vi "Rollback Transaction.vi"(8 "error in":errorcluster, 11 "DB-SQLite in":refnum<class "DB-SQLite.lvclass">) -> (0 "error out":errorcluster, 3 "DB-SQLite out":refnum<class "DB-SQLite.lvclass">)   [LabVIEW 2022 SP3, in "hse-db-sqlite.lvlib" / "DB-SQLite.lvclass"]
doc: "Rollback the active transaction.\n\n____\nHAMPEL SOFTWARE ENGINEERING v1.4.0 (2023-12-19 09:52)"
uses:
  DB-SQLite.lvclass
  DB-SQLite.lvclass/DB-SQLite.ctl
  <vilib>/drjdpowell/SQLite Library/Transaction Helpers/Transaction.lvlib
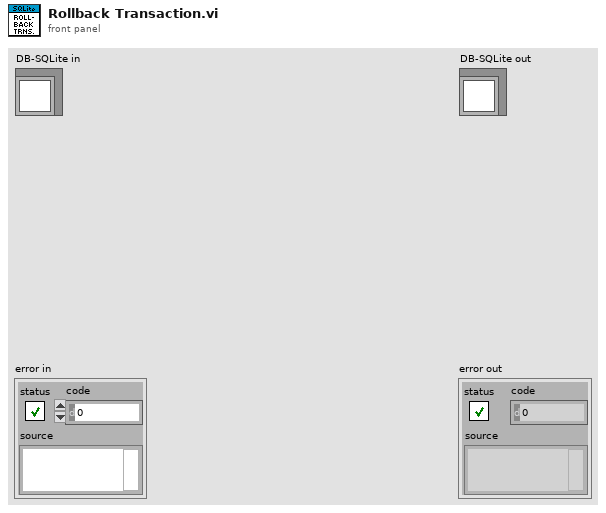
[diagram p1: front panel]
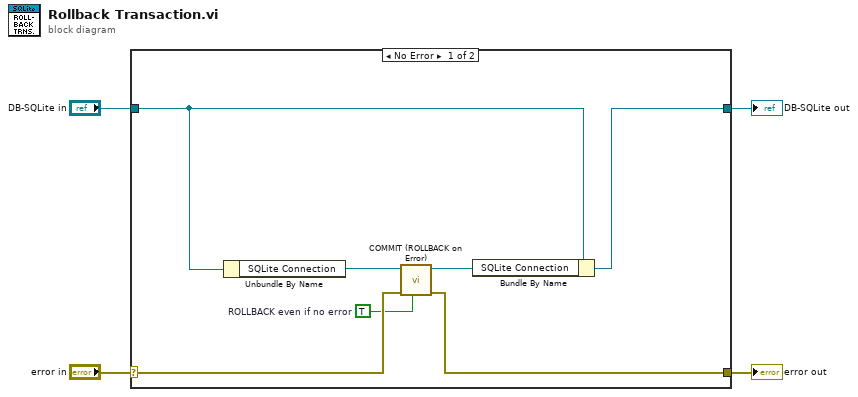
[diagram p0: block diagram]
diagram:
  n1 = case shown="No Error" "error in" {
    selector: "error in" -> [w9 w13]
    tunnel: [w6 w13] -> w3
    tunnel: [w10 w12] -> w1
    tunnel: "DB-SQLite in" -> [w11 w12]
    frame No Error {
      w5 = TRUE  # ROLLBACK even if no error
      n2 = Unbundle By Name(w11) -> ("SQLite Connection"=w8:refnum<class "Connection.lvclass">)
      n3 = call <vilib>:"COMMIT (ROLLBACK on Error).vi"("ROLLBACK even if no error"=w5, "error in (no error)"=w9, "SQLite Connection in"=w8) -> ("error out"=w6:errorcluster, "SQLite Connection"=w7:refnum<class "Connection.lvclass">)  [unwired: 7 in]
      n4 = Bundle By Name(cluster=w11, "SQLite Connection"=w7) -> (w10:refnum<class "DB-SQLite.lvclass">)
    }
    frame Error {
    }
  }
  "error out" <- w3
  "DB-SQLite out" <- w1
